vi "Test Errors Are Logged.vi"(8 "error in (no error)":errorcluster, 11 "Test Case In":refnum<class "Error Handler Tests.lvclass">) -> (0 "error out":errorcluster, 3 "Test Case Out":refnum<class "Error Handler Tests.lvclass">)   [LabVIEW 2020, in "Error Handler Tests.lvclass"]
uses:
  Error Handler Tests.lvclass
  C:/Program Files (x86)/National Instruments/LabVIEW 2020/vi.lib/Astemes/LUnit/Test Case.lvclass
  <vilib>/Utility/sysdir.llb/System Directory Type.ctl
  <vilib>/Astemes/LUnit/Test Case.lvclass/Test Case.ctl
  f68d6c05-d397-4b87-971a-b851a749559a.vi
  <vilib>/Astemes/LUnit/Core/LUnit Test Case/Private/Append Pass Result.vi
  <vilib>/Astemes/LUnit/Core/LUnit Test Case/Private/Append Fail Result.vi
  f68d6c05-d397-4b87-971a-b851a749559a.vi/9c5d11cd-9439-4240-a1ee-d9baace9c924.vi
  <vilib>/Astemes/LUnit/Core/LUnit Test Case/Private/Run In UI.vi
  <vilib>/Utility/error.llb/Clear Errors.vi
  source/User Interface/Process/Process.lvclass
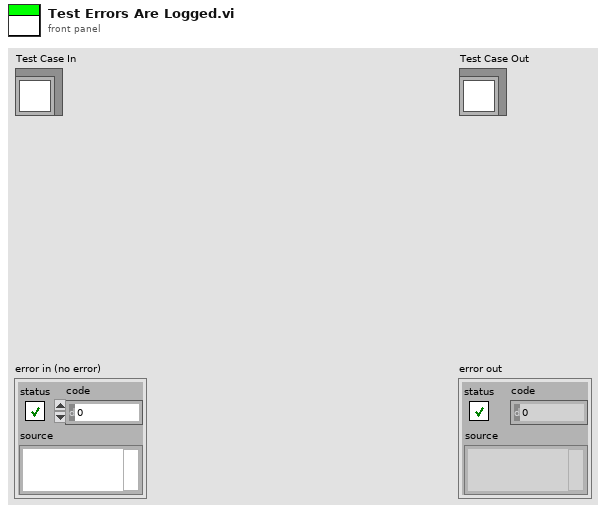
[diagram p1: front panel]
types:
  T1 = typedef "System Directory Type.ctl" = i32
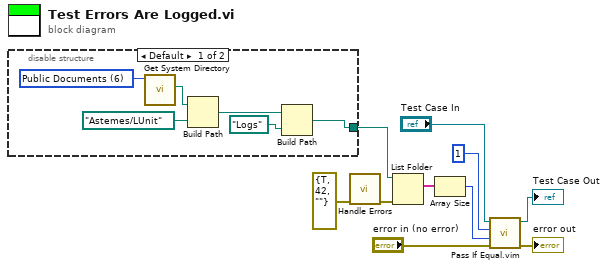
[diagram p0: block diagram]
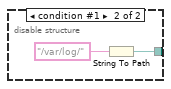
[diagram p2: hidden frame]
diagram:
  n1 = disable-structure shown="Default" {
    disable-tunnel: [w16 w17] -> w6
    frame condition #0 (active) {
      w11 = T1 6 items=["User Home"=0, "User Desktop"=1, "User Documents"=2, "User Application Data"=3, "User Preferences"=4, "User Temporary"=5, "Public Documents"=6, "Public Application Data"=7, "Public Preferences"=8, "Public Cache"=13, "System Core Libraries"=9, "System Installed Libraries"=10, "Application Files"=11, "Boot Volume Root"=12] ("system directory type")
      n2 = call <vilib>:"Get System Directory.vi"("system directory type"=w11) -> ("system directory"=w13:path)  [unwired: 10 in]
      n3 = Build Path(base path=w13, name or relative path=path "Astemes/LUnit") -> (appended path=w14:path)
      n4 = Build Path(base path=w14, name or relative path=path "Logs") -> (appended path=w16:path)
    }
    frame condition #1 {
      n5 = String To Path(string="/var/log/") -> (path=w17:path)
    }
  }
  n6 = call "Handle Errors.vi"("error in (no error)"=errorcluster {"status"=TRUE, "code"=42, "source"=""}) -> ("error out"=w2:errorcluster)  [unwired: 10 in]
  n7 = List Folder(path=w6, error in=w2) -> (filenames=w5:string[])  [unwired: 2 in, 3 out]
  n8 = Array Size(array=w5) -> (size(s)=w4:i32)
  n9 = call "Pass If Equal.vim"("error in (no error)"="error in (no error)", "Actual"=w4, "Expected"=1 ("size(s)"), "LUnit Test Case In"="Test Case In") -> ("error out"=→"error out":errorcluster, "LUnit Test Case Out"=→"Test Case Out":refnum<class "Error Handler Tests.lvclass">)  [unwired: 6 in]
